vi "FTW-JSON-Object-SetElement-String.vi"(0 "JSON Object":refnum<data-value>, 5 "Key":string, 7 "Value":string, 11 "error in":errorcluster) -> (4 "JSON Object out":refnum<data-value>, 15 "error out":errorcluster)   [LabVIEW 2015]
uses:
  core/FTW-JSON-Core-Structure.ctl
  error/FTW-ERR-ThrowError.vi
  error/FTW-ERR-CallChain.vi
  error/FTW-ERR-NoErrorConstant.vi
  string/FTW-STR-ReplaceWhitespace.vi
  string/FTW-STR-Array-Delimit.vi
  error/FTW-ERR-Clear.vi
  regex/FTW-Regex-ReplaceAll.vi
panel:
  # "Inputs"
  # "Outputs"
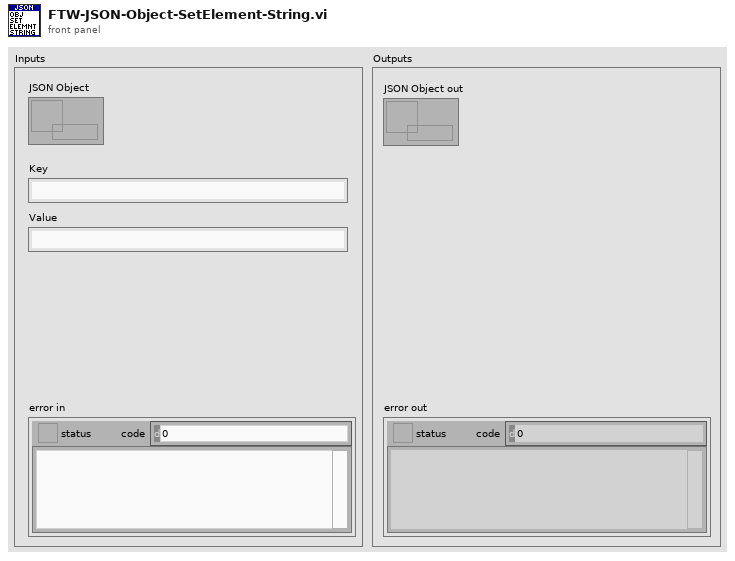
[diagram p1: front panel]
types:
  T1 = typedef "FTW-JSON-Core-Structure.ctl" = cluster{"JSON Object":i64, "Encoding Flags":i64, "Decoding Flags":i64}
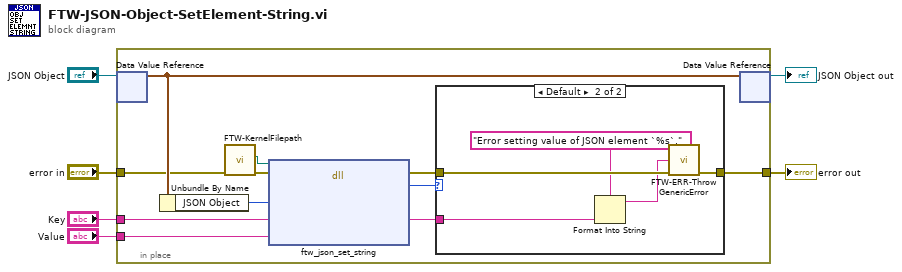
[diagram p0: block diagram]
diagram:
  n1 = in-place {
    in-place-border: "error in" -> [w9]
    in-place-border: [w10] -> w4
    in-place-border: "Key" -> [w17]
    in-place-border: "Value" -> [w14]
    n2 = in-place-dvr #1("JSON Object") -> (w16:T1)  [unwired: 1 out]
    n3 = Unbundle By Name(w16) -> ("JSON Object"=w15:i64)
    n4 = call "FTW-KernelFilepath.vi"("error in"=w9) -> ("error out"=w8:errorcluster, "Library Filepath"=w7:path)  [unwired: 8 in, 1 out]
    n5 = dll-call lib="?" fn="ftw_json_set_string"(path in=w7, error in=w8, "JSON Object Pointer"=w15, "Key"=w17, "New Value"=w14) -> (error out=w12:errorcluster, "Return Value"=w13:i64, "Key"=w11:string)  [unwired: 3 in, 1 out]
    n6 = case shown="Default" w13 {
      tunnel: w12 -> [w18 w23]
      tunnel: w11 -> [_ w20]
      tunnel: [w18 w22] -> w10
      frame 0 {
      }
      frame Default {
        n7 = Format Into String(format string="Error setting value of JSON element `%s`.", w20) -> (resulting string=w19:string)  [unwired: 2 in, 1 out]
        n8 = call "FTW-ERR-ThrowGenericError.vi"("Error Message"=w19, "error in"=w23) -> ("error out"=w22:errorcluster)  [unwired: 13 in]
      }
    }
    n9 = in-place-dvr #1(w16) -> (→"JSON Object out":refnum<data-value>)  [unwired: 1 out]
  }
  "error out" <- w4
